vi "Reorder Chromosome  After Makespan Calculation.vi"(9 "Number Of  Jobs":i32, 10 "Number Of Machines":i32, 11 "Gannt Chart In":T1[][](array[typedef])) -> (3 "Reordered Chromosome":u16[](array[numeric]))   [LabVIEW 2013, in "GanntChart.lvclass"]
uses:
  GanntChart.lvclass
  Controls/GanntChart_Element.ctl
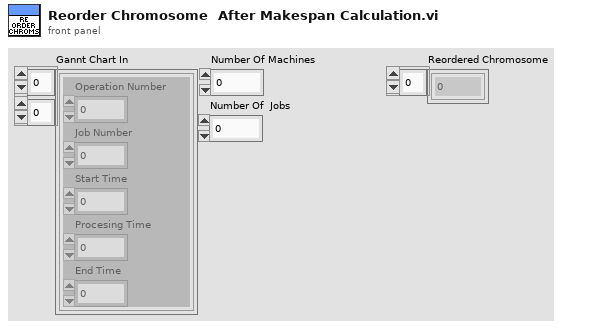
[diagram p1: front panel]
types:
  T1 = typedef "GanntChart_Element.ctl" = cluster{"Operation Number":i32, "Job Number":i32, "Start Time":i32, "Procesing Time":u16, "End Time":i32}
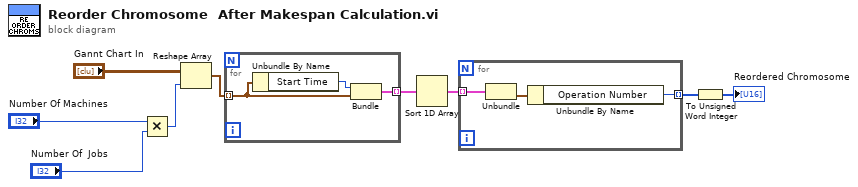
[diagram p0: block diagram]
diagram:
  n1 = Multiply(x="Number Of Machines", y="Number Of  Jobs") -> (x*y=w6:i32)
  n2 = Reshape Array("Gannt Chart In", w6) -> (w5:T1[])
  n3 = for {
    tunnel: w5 -> [w11] mode=indexing
    tunnel: [w10] -> w4 mode=indexing
    n4 = Unbundle By Name(w11) -> ("Start Time"=w12:i32)
    n5 = Bundle("Start Time"=w12, w11) -> (w10:cluster{"Start Time":i32, T1})  [unwired: 1 in]
  }
  n6 = Sort 1D Array(array=w4) -> (sorted array=w3:cluster{"Start Time":i32, T1}[])
  n7 = for {
    tunnel: w3 -> [w15] mode=indexing
    tunnel: [w13] -> w2 mode=indexing
    n8 = Unbundle(w15) -> (w14:T1)  [unwired: 1 out]
    n9 = Unbundle By Name(w14) -> ("Operation Number"=w13:i32)
  }
  n10 = To Unsigned Word Integer(number=w2) -> (unsigned 16bit integer=→"Reordered Chromosome":u16[])
